vi "LNA Stopped.vi"(8 "error in (no error)":errorcluster, 11 "Client Controller in":refnum<class "Client Controller.lvclass">) -> (0 "error out":errorcluster, 3 "Client Controller out":refnum<class "Client Controller.lvclass">)   [LabVIEW 2013, in "Client Controller.lvlib" / "Client Controller.lvclass"]
uses:
  Client Controller.lvclass
  Client Controller.lvclass/Client Controller.ctl
  <vilib>/ActorFramework/Actor/Actor.lvclass/Actor.ctl
  <vilib>/ActorFramework/Message Enqueuer/Message Enqueuer.lvclass/Message Enqueuer.ctl
  <vilib>/ActorFramework/Message Enqueuer/Init from Existing Queue.vi
  <vilib>/ActorFramework/Message Enqueuer/Enqueue.vi
  <vilib>/ActorFramework/Message Priority Queue/Priority Enqueue.vi
  <vilib>/ActorFramework/Message Enqueuer/Message Enqueuer.lvclass
  Messages/Negotiate Server Connection Msg/Negotiate Server Connection Msg.lvclass
  <vilib>/ActorFramework/Actor/Actor.lvclass
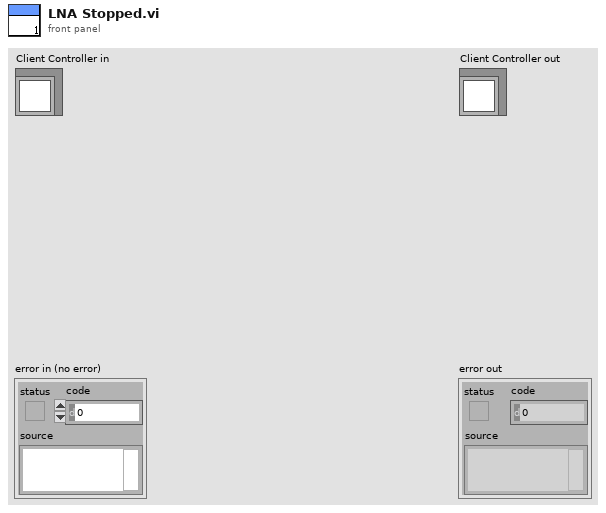
[diagram p1: front panel]
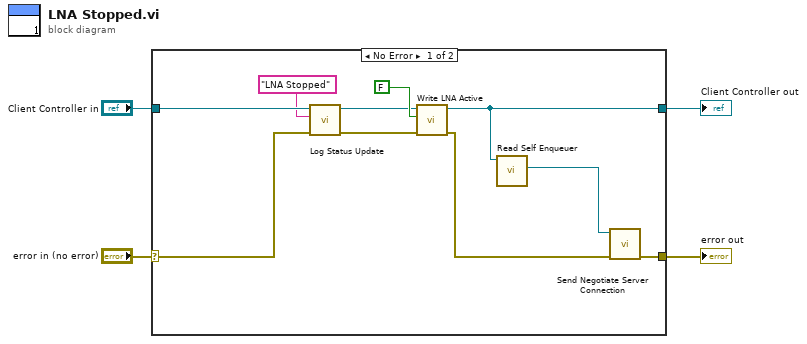
[diagram p0: block diagram]
diagram:
  n1 = case shown="No Error" "error in (no error)" {
    selector: "error in (no error)" -> [w6 w16]
    tunnel: [w5 w16] -> w3
    tunnel: [w13 w15] -> w1
    tunnel: "Client Controller in" -> [w11 w15]
    frame No Error {
      n2 = call-dynamic "Log Status Update.vi"("error in (no error)"=w6, "String"="LNA Stopped", "Controller in"=w11) -> ("error out"=w8:errorcluster, "Controller out"=w10:refnum<class "Client Controller.lvclass">)  [unwired: 7 in]
      n3 = call "Write LNA Active.vi"("error in (no error)"=w8, "LNA Active?"=FALSE, "Client Controller in"=w10) -> ("error out"=w9:errorcluster, "Client Controller out"=w13:refnum<class "Client Controller.lvclass">)  [unwired: 7 in]
      n4 = call <vilib>:"Read Self Enqueuer.vi"("Actor"=w13) -> ("Self Enqueuer"=w12:refnum<class "Message Enqueuer.lvclass">)  [unwired: 10 in]
      n5 = call "Send Negotiate Server Connection.vi"("error in (no error)"=w9, "Message Enqueuer"=w12) -> ("error out"=w5:errorcluster)  [unwired: 8 in, 1 out]
    }
    frame Error {
    }
  }
  "error out" <- w3
  "Client Controller out" <- w1
